vi "NF LI56xx dvr MATH normalize.vi"(8 "error in":errorcluster caption="error in (no error)" {"code" format="%.0x"}, 9 "Read(F)":bool, 10 "set normalize calculation format":enum16{"DB", "PCNT", "PCFS"}(ring), 11 "VISA resource name":refnum<visa-resource-name>) -> (0 "error out":errorcluster {"code" format="%.0x"}, 2 "query normalize calculation format":string, 3 "VISA resource name copy":refnum<visa-resource-name>)   [LabVIEW 2019]
doc: "Sets/queries the normalize calculation format. \nDisplay and output of normalize results also requires enabling normalize calculation with the :CALCulate5:MATH NORM command. \nReference values are set with \n :CALCulate:MATH:CURRent[:LEVel] command (current) and\n :CALCulate:MATH:VOLTage[:LEVel] command (voltage)"
panel:
  out "query unit name":string
  in  "set unit name":string
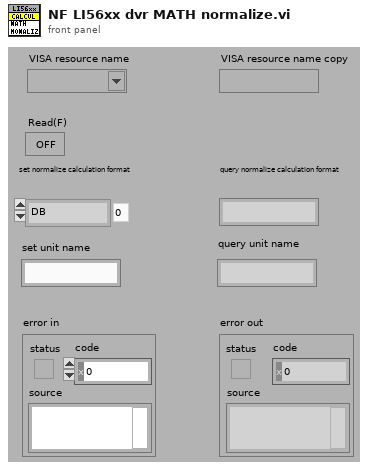
[diagram p1: front panel]
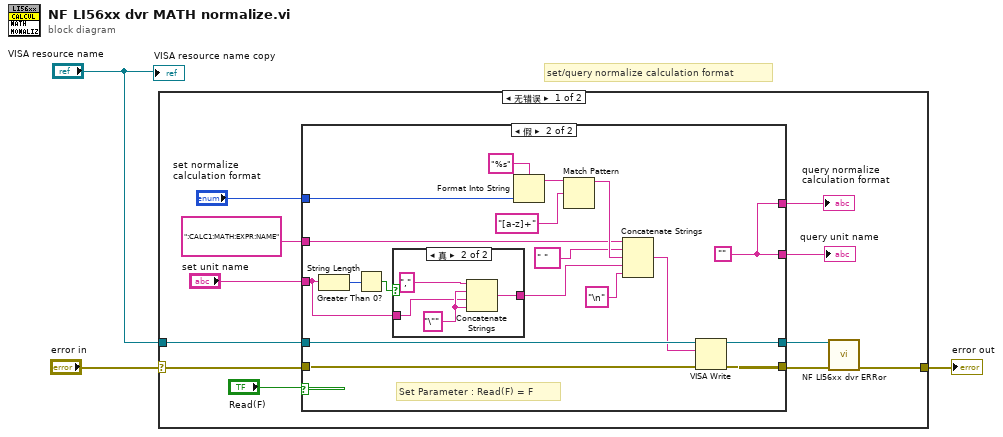
[diagram p0: block diagram]
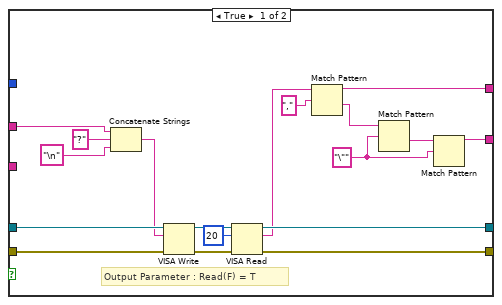
[diagram p2: hidden frame]
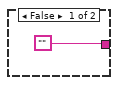
[diagram p3: hidden frame]
diagram:
  # "set/query normalize calculation format"
  n1 = case shown="无错误" "error in" {
    selector: "error in" -> [w13 w56]
    tunnel: [w8 w56] -> w3
    tunnel: "VISA resource name" -> [w12 _]
    frame No Error {
      n2 = case shown="假" "Read(F)" {
        tunnel: w12 -> [w32 w50]
        tunnel: [w29 w47] -> w10
        tunnel: [w28 w48] -> w9
        tunnel: w13 -> [w27 w49]
        tunnel: "set normalize calculation format" -> [_ w44]
        tunnel: ":CALC1:MATH:EXPR:NAME" ("•¶Žš—ñ") -> [w22 w40]
        tunnel: "set unit name" -> [_ w36]
        tunnel: [w15 w35] -> w5
        tunnel: [w19 w35] -> w4
        frame True {
          w16 = "\"" ("³K\\»")
          # "Output Parameter : Read(F) = T"
          n3 = Concatenate Strings(w22, "?" ("Œ`Ž®•¶Žš—ñ"), "\n" ("Œ`Ž®•¶Žš—ñ")) -> (w24:string)
          n4 = VISA Write(VISA resource name=w32, write buffer=w24, error in (no error)=w27) -> (VISA resource name out=w30:refnum<visa-resource-name>, error out=w31:errorcluster)  [unwired: 1 out]
          n5 = VISA Read(VISA resource name=w30, byte count=u32 20 ("バイトカウント（0）"), error in (no error)=w31) -> (VISA resource name out=w29:refnum<visa-resource-name>, read buffer=w21:string, error out=w28:errorcluster)  [unwired: 1 out]
          n6 = Match Pattern(string=w21, regular expression="," ("³K\\»")) -> (before substring=w19:string, after substring=w18:string)  [unwired: 1 in, 2 out]
          n7 = Match Pattern(string=w18, regular expression=w16) -> (after substring=w17:string)  [unwired: 1 in, 3 out]
          n8 = Match Pattern(string=w17, regular expression=w16) -> (before substring=w15:string)  [unwired: 1 in, 3 out]
        }
        frame False {
          w35 = ""
          # "Set Parameter : Read(F) = F"
          n9 = String Length(string=w36) -> (length=w39:i32)
          n10 = Greater Than 0?(x=w39) -> (x > 0?=w38:bool)
          n11 = case shown="真" w38 {
            tunnel: ["" w55] -> w34
            tunnel: w36 -> [_ w53]
            frame False {
            }
            frame True {
              w54 = "\"" ("•¶Žš—ñ")
              n12 = Concatenate Strings("," ("•¶Žš—ñ"), w54, w53, w54) -> (w55:string)
            }
          }
          n13 = Format Into String(format string="%s", w44) -> (resulting string=w43:string)  [unwired: 2 in, 1 out]
          n14 = Match Pattern(string=w43, regular expression="[a-z]+") -> (before substring=w42:string)  [unwired: 1 in, 3 out]
          n15 = Concatenate Strings(w40, " ", w42, w34, "\n" ("Œ`Ž®•¶Žš—ñ")) -> (w46:string)
          n16 = VISA Write(VISA resource name=w50, write buffer=w46, error in (no error)=w49) -> (VISA resource name out=w47:refnum<visa-resource-name>, error out=w48:errorcluster)  [unwired: 1 out]
        }
      }
      "query normalize calculation format" <- w4
      "query unit name" <- w5
      n17 = call "NF LI56xx dvr ERRor.vi"("VISA resource name"=w10, "error in (no error)"=w9) -> ("error out"=w8:errorcluster)  [unwired: 10 in, 3 out]
    }
    frame Error {
    }
  }
  "error out" <- w3
  "VISA resource name copy" <- "VISA resource name"
